vi "Flush Client Handles.vi"(8 "error in (no error)":errorcluster, 11 "REST Client in":refnum<class "REST Client_JKI.lvclass">) -> (0 "error out":errorcluster, 3 "REST Client out":refnum<class "REST Client_JKI.lvclass">)   [LabVIEW 2018, in "REST Client.lvlib" / "REST Client_JKI.lvclass"]
doc: "Destroy REST client reference."
uses:
  REST Client_JKI.lvclass
  REST Client_JKI.lvclass/REST Client_JKI.ctl
  <vilib>/httpClient/LabVIEWHTTPClient.lvlib
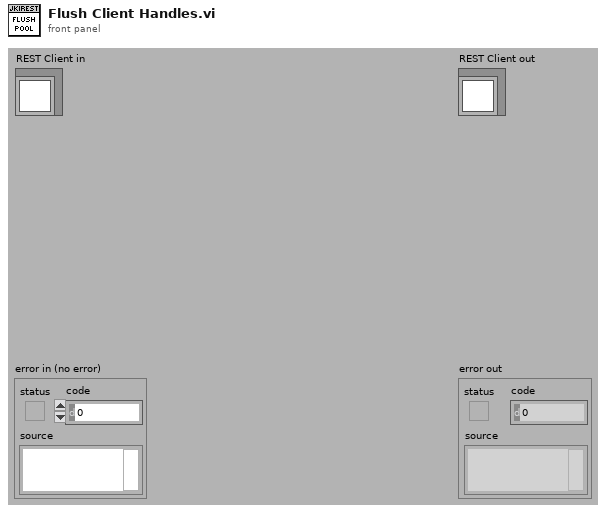
[diagram p1: front panel]
types:
  T1 = typedef "LabVIEWHTTPClient.lvlib/ClientHandle.ctl" = refnum<k1>
  T2 = typedef "REST Client.lvlib/REST Client.lvclass/HTTP Header.ctl" = cluster{"header":string, "value":string}
  T3 = cluster{"client handle out":T1, "Default Headers ([JSON])":T2[]}[]
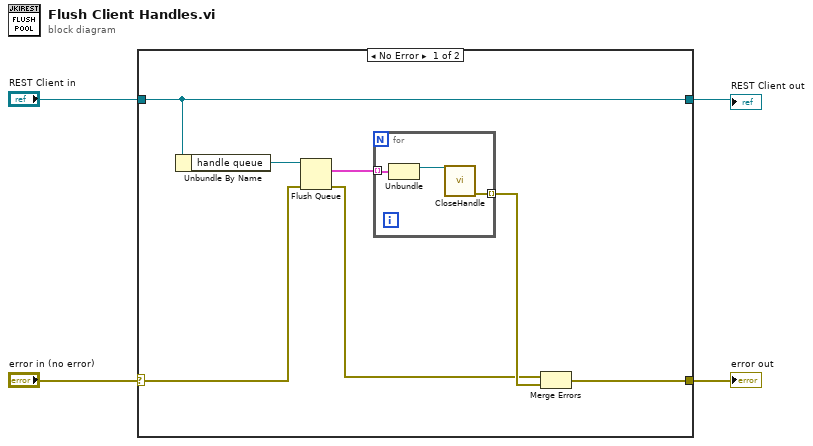
[diagram p0: block diagram]
diagram:
  n1 = case shown="No Error" "error in (no error)" {
    selector: "error in (no error)" -> [w6 w15]
    tunnel: "REST Client in" -> [w7 w16]
    tunnel: [w9 w15] -> w3
    tunnel: [w7 w16] -> w1
    frame No Error {
      n2 = Unbundle By Name(w7) -> ("handle queue"=w11:refnum<queue>)
      n3 = Flush Queue(queue=w11, error in (no error)=w6) -> (remaining elements=w10:T3, error out=w5:errorcluster)  [unwired: 1 out]
      n4 = for {
        tunnel: w10 -> [w13] mode=indexing
        tunnel: [w14] -> w8 mode=indexing
        n5 = Unbundle(w13) -> ("client handle out"=w12:T1)  [unwired: 1 out]
        n6 = call <vilib>:"CloseHandle.vi"("client handle"=w12) -> ("error out"=w14:errorcluster)  [unwired: 14 in]
      }
      n7 = Merge Errors(w5, w8) -> (w9:errorcluster)
    }
    frame Error {
    }
  }
  "error out" <- w3
  "REST Client out" <- w1
